vi "4Pi 4Pi Modes - Select Modes - BAK.vi"() -> ()   [LabVIEW 2016]
uses:
  4Pi 4Pi Modes - Controls/4Pi 4Pi Modes - Mirror Modes.ctl
  <vilib>/Utility/miscctls.llb/LVPointTypeDef.ctl
  Hardware Configuration/Hardware Configuration Controls/Standard Action.ctl
  4Pi 4Pi Modes - Controls/4Pi 4Pi Modes - Standard Action.ctl
  <userlib>/BMC/BMC.lvlib
panel:
  out "error out":errorcluster
  in  "Mirror Modes":T1
  in  "Flags":string
  in  "Change Modes":bool
  in  "Help":bool
  in  "Control mode":string(combo)="Single"
  in  "DM index":string(combo)="0"
  out "standard output":string
  out "standard error":string
  in  "Calling VI Ref":refnum<vi>
  in  "Exit":bool
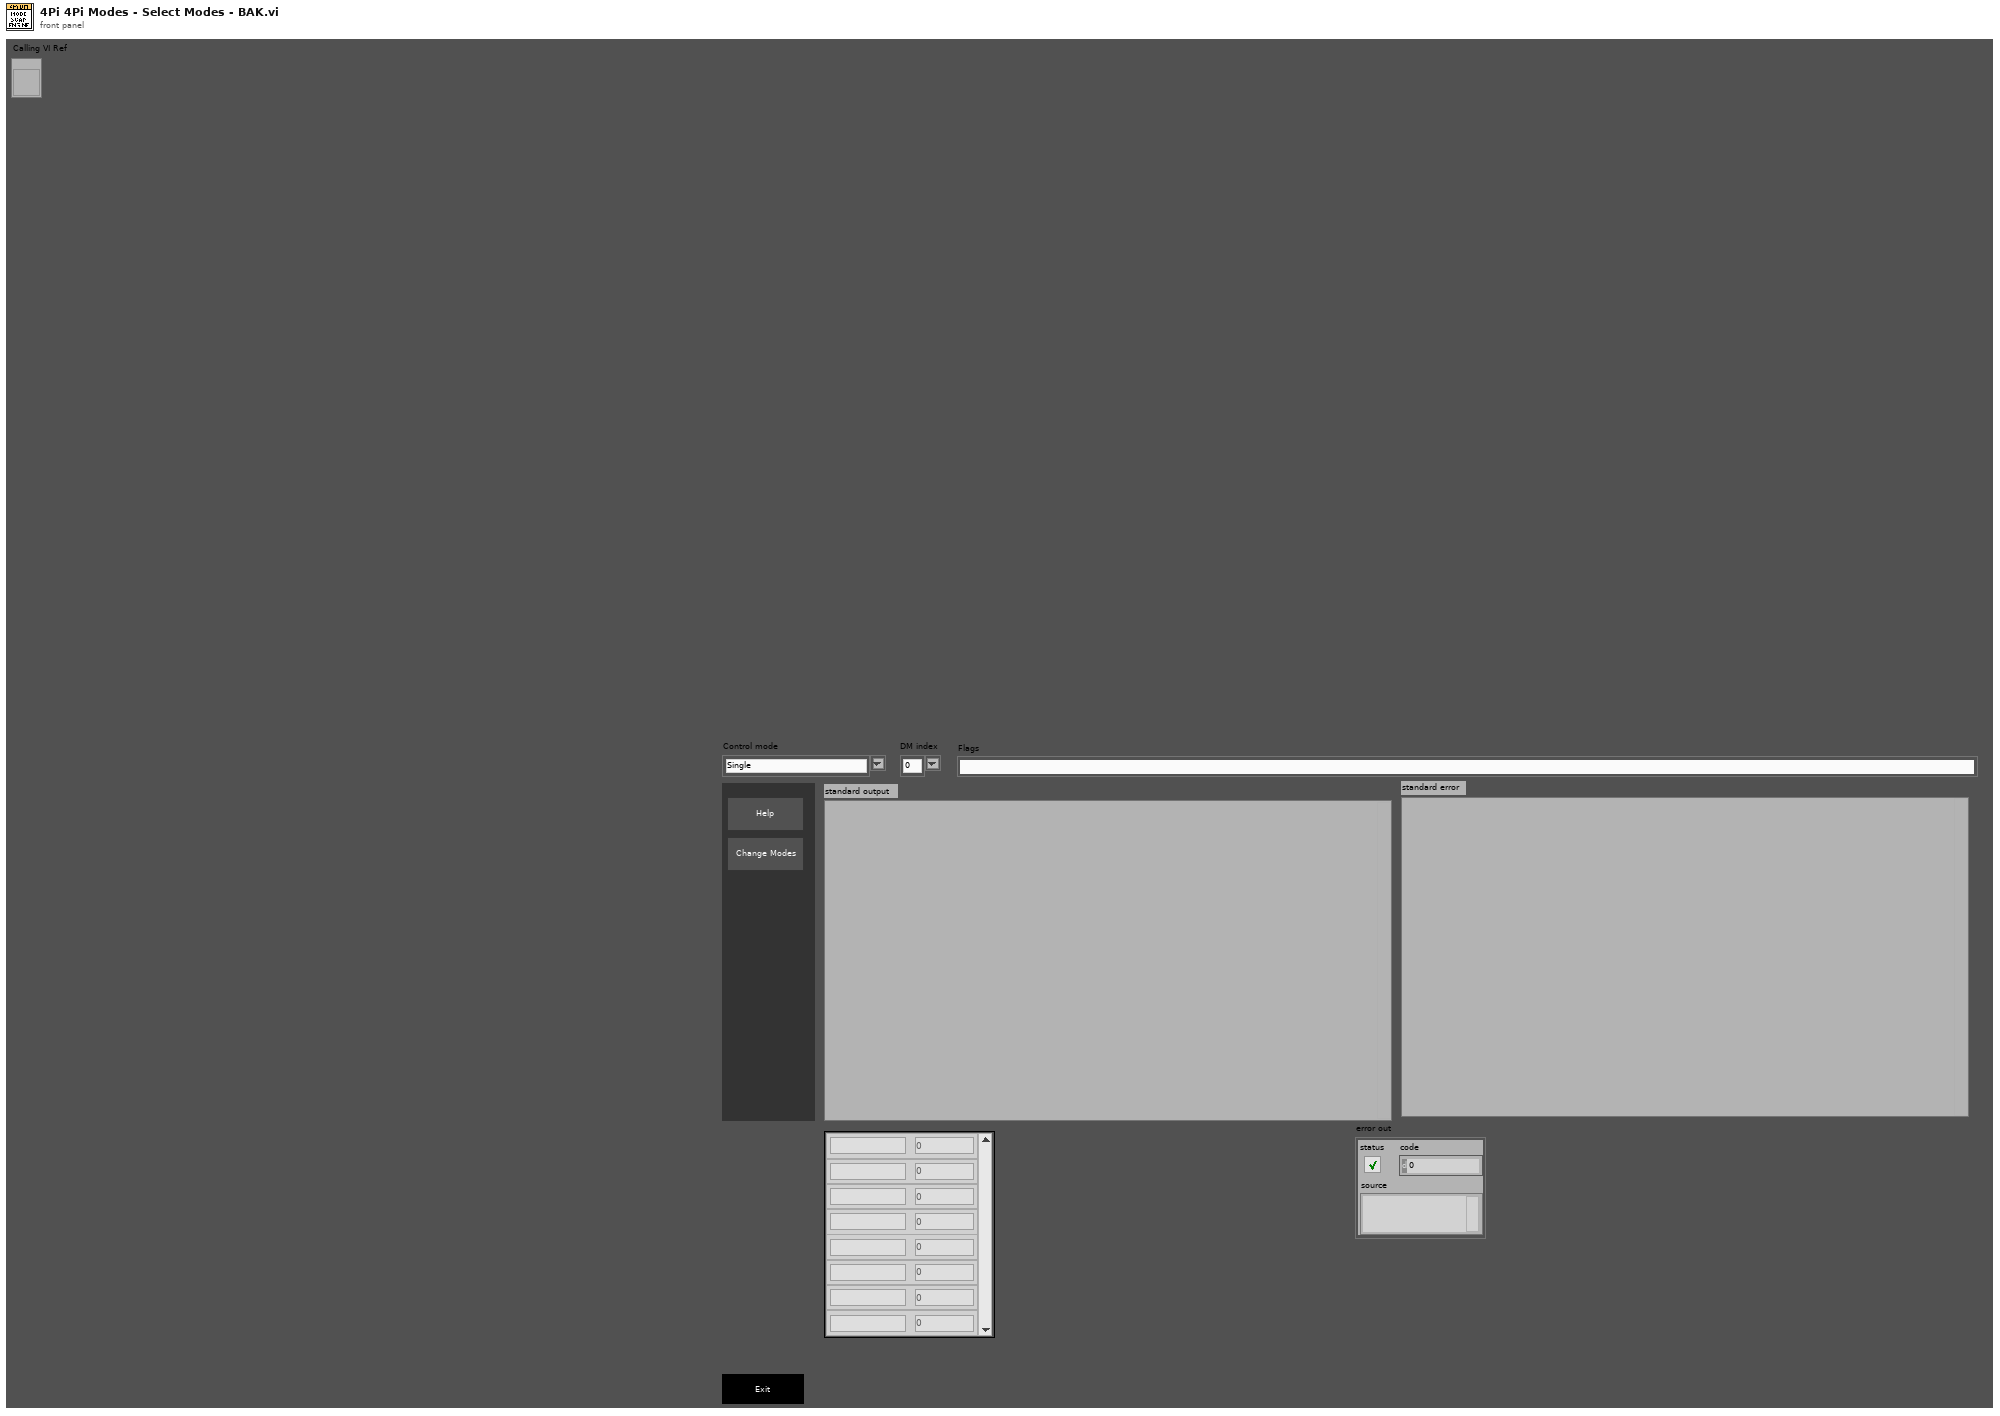
[diagram p1: front panel]
types:
  T1 = typedef "4Pi 4Pi Modes - Mirror Modes.ctl" = cluster{"Mode":string, "Amplitude":dbl}[]
  T2 = enum16{"Always On", "Always Off", "Off While Running"}
  T3 = typedef "LVPointTypeDef.ctl" = cluster{"Horizontal":i16, "Vertical":i16}
  T4 = typedef "LVRectTypeDef.ctl" = cluster{"Left":i16, "Top":i16, "Right":i16, "Bottom":i16}
  T5 = typedef "LVBoundsTypeDef.ctl" = cluster{"Width":u32, "Height":u32}
  T6 = typedef "Standard Action.ctl" = enum16{"Read", "Write"}
  T7 = typedef "4Pi 4Pi Modes - Standard Action.ctl" = enum16{"Read", "Write"}
  T8 = cluster{"type":i16, "ID":i16, "size":i32, "lutName":u64, "priv":u64}[]
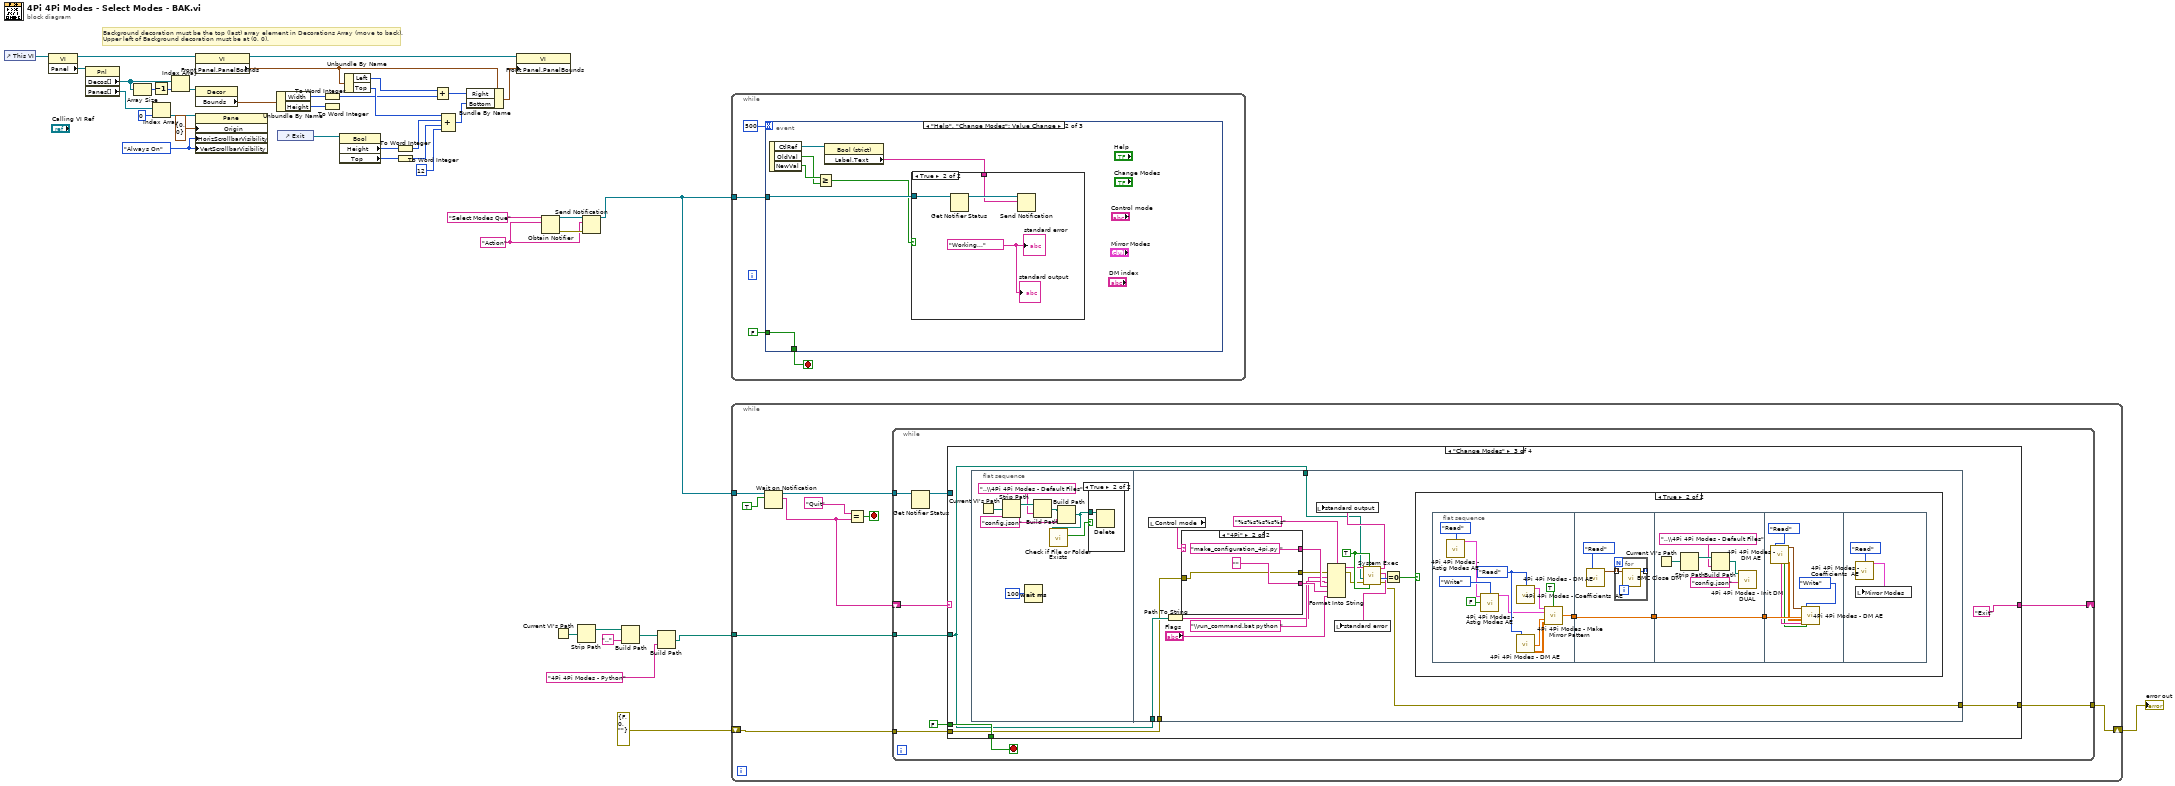
[diagram p0: block diagram]
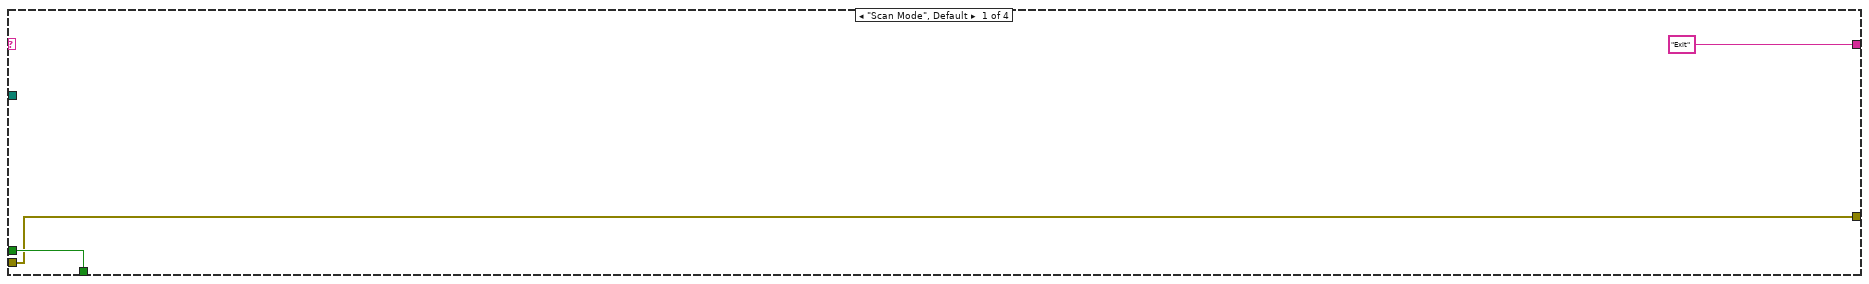
[diagram p2: hidden frame]
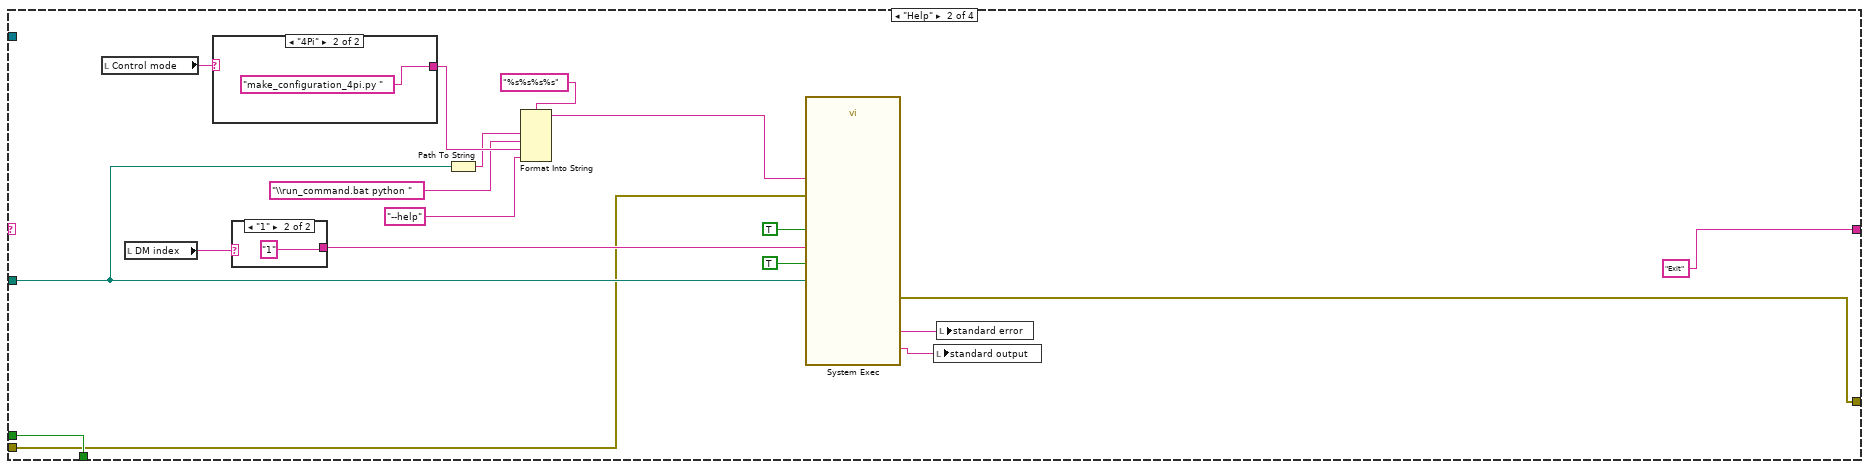
[diagram p3: hidden frame]
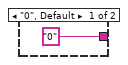
[diagram p4: hidden frame]
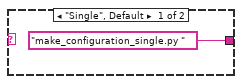
[diagram p5: hidden frame]
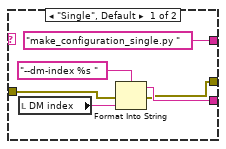
[diagram p8: hidden frame]
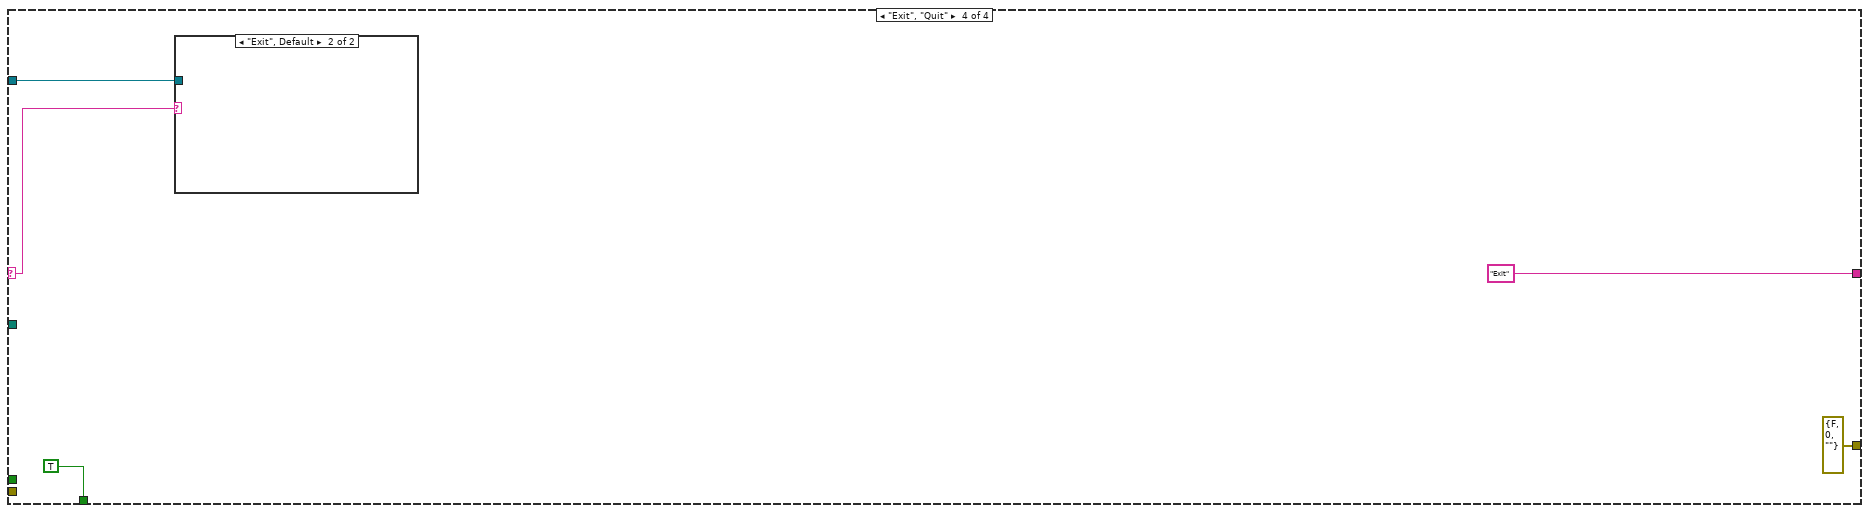
[diagram p9: hidden frame]
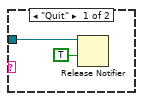
[diagram p10: hidden frame]
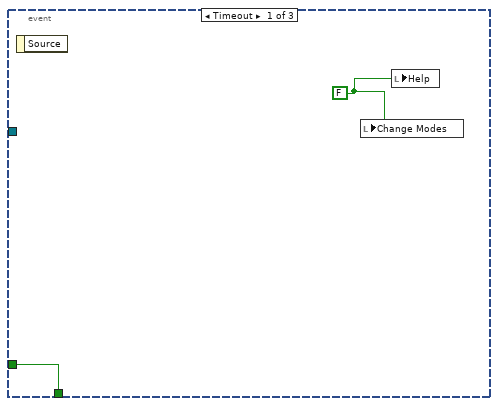
[diagram p11: hidden frame]
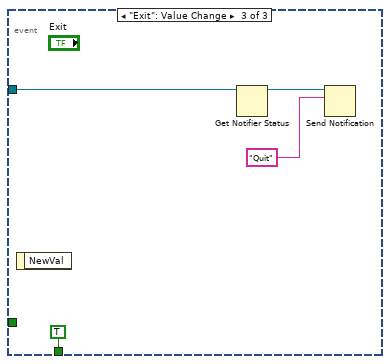
[diagram p13: hidden frame]
diagram:
  w9 = "Action" ("name (unnamed)")
  w25 = T2."Always On" ("Vertical Scrollbar Visibility")
  # "Background decoration must be the top (last) array element in Decorations Array (move to back).\nUpper left of Background decoration must be at (0, 0)."
  n1 = control-ref of="This VI"() -> (w17:refnum<vi>)
  n2 = property class="VI"(reference=w17) -> (reference out=w26:refnum<vi>, "Panel"=w18:refnum<vi>)  [unwired: 1 in, 1 out]
  n3 = property class="Pnl"(reference=w18) -> ("Decos[]"=w16:refnum<vi>[], "Panes[]"=w22:refnum<vi>[])  [unwired: 1 in, 2 out]
  n4 = Array Size(array=w16) -> (size(s)=w14:i32)
  n5 = Decrement(x=w14) -> (x-1=w15:i32)
  n6 = Index Array(array=w22, index=0) -> (element=w21:refnum<vi>)
  n7 = Index Array(array=w16, index=w15) -> (element=w24:refnum<vi>)
  n8 = property class="VI"(reference=w26) -> (reference out=w28:refnum<vi>, "Front Panel.PanelBounds"=w29:T4)  [unwired: 1 in, 1 out]
  n9 = property class="Decor"(reference=w24) -> ("Bounds"=w27:T5)  [unwired: 1 in, 2 out]
  n10 = property class="Pane"(reference=w21, "Origin"=T3 {"Horizontal"=0, "Vertical"=0}, "HorizScrollbarVisibility"=w25, "VertScrollbarVisibility"=w25) -> ()  [unwired: 1 in, 2 out]
  n11 = Unbundle By Name(w27) -> ("Width"=w32:u32, "Height"=w35:u32)
  n12 = control-ref of="Exit"() -> (w19:refnum<vi>)
  n13 = To Word Integer(number=w32) -> (16bit integer=w34:i16)
  n14 = To Word Integer(number=w35) -> ()  [unwired: 1 out]
  n15 = property class="Bool"(reference=w19) -> ("Height"=w37:u32, "Top"=w38:i32)  [unwired: 1 in, 2 out]
  n16 = Unbundle By Name(w29) -> ("Left"=w31:i16, "Top"=w42:i16)
  n17 = To Word Integer(number=w37) -> (16bit integer=w40:i16)
  n18 = To Word Integer(number=w38) -> (16bit integer=w41:i16)
  n19 = Add(x=w31, y=w34) -> (x+y=w33:i16)
  n20 = Compound Arithmetic op=ADD(w42, w40, w41, i16 12 ("y")) -> (w36:i16)
  n21 = Bundle By Name(cluster=w29, "Right"=w33, "Bottom"=w36) -> (w30:T4)
  n22 = property class="VI"(reference=w28, "Front Panel.PanelBounds"=w30) -> ()  [unwired: 1 in, 2 out]
  n23 = Obtain Notifier(name (unnamed)="Select Modes Que", notification data type=w9) -> (notifier out=w11:refnum<notifier>, error out=w12:errorcluster)  [unwired: 2 in, 1 out]
  n24 = Current VI's Path() -> (path=w7:path)
  n25 = Strip Path(path=w7) -> (stripped path=w6:path)  [unwired: 1 out]
  n26 = Send Notification(notification=w9, notifier=w11, error in (no error)=w12) -> (notifier out=w10:refnum<notifier>)  [unwired: 1 out]
  n27 = Build Path(base path=w6, name or relative path="..") -> (appended path=w4:path)
  n28 = Build Path(base path=w4, name or relative path="4Pi 4Pi Modes - Python") -> (appended path=w3:path)
  n29 = while {
    tunnel: w10 -> [w45]
    stop <- w43 stop-if-true
    n30 = event shown="[1] \"Help\", \"Change Modes\": Value Change" {
      selector: _ -> [_ _ _]
      dyn-events: _ -> [_ _ _]
      timeout: 500 -> [_ _ _]
      tunnel: w45 -> [_ w55 w62]
      tunnel: [w48 w54 TRUE] -> w43
      tunnel: FALSE -> [w48 w54 _]
      event Timeout {
        w47 = FALSE
        n31 = event-data() -> ()  [unwired: 1 in, 1 out]
        n32 = local write "Change Modes"(w47) -> ()
        n33 = local write "Help"(w47) -> ()
      }
      event "Help", "Change Modes": Value Change {
        n34 = event-data() -> ("CtlRef"=w53:refnum<vi>, "OldVal"=w50:bool, "NewVal"=w51:bool)  [unwired: 1 in]
        n35 = Greater Or Equal?(x=w51, y=w50) -> (x >= y?=w49:bool)
        n36 = property class="Bool (strict)"(reference=w53) -> ("Label.Text"=w52:string)  [unwired: 1 in, 2 out]
        n37 = case shown="True" w49 {
          tunnel: w55 -> [_ w58]
          tunnel: w52 -> [_ w56]
          frame False {
          }
          frame True {
            w57 = "Working..." ("standard error")
            n38 = Get Notifier Status(notifier=w58) -> (notifier out=w59:refnum<notifier>)  [unwired: 1 in, 4 out]
            n39 = Send Notification(notification=w56, notifier=w59) -> ()  [unwired: 1 in, 2 out]
            "standard error" <- w57
            "standard output" <- w57
          }
        }
      }
      event "Exit": Value Change {
        n40 = event-data() -> ()  [unwired: 1 in, 1 out]
        n41 = Get Notifier Status(notifier=w62) -> (notifier out=w63:refnum<notifier>)  [unwired: 1 in, 4 out]
        n42 = Send Notification(notification="Quit", notifier=w63) -> ()  [unwired: 1 in, 2 out]
      }
    }
  }
  n43 = while {
    tunnel: w10 -> [w72]
    tunnel: w3 -> [w66]
    shift-right: [w65] -> w1
    shift-left: errorcluster {"status"=FALSE, "code"=0, "source"=""} ("error in") -> [w64]
    stop <- w69 stop-if-true
    n44 = Wait on Notification(notifier=w72, ignore previous (F)=TRUE) -> (notifier out=w70:refnum<notifier>, notification=w67:string)  [unwired: 2 in, 2 out]
    n45 = Equal?(x="Quit" ("name (unnamed)"), y=w67) -> (x = y?=w69:bool)
    n46 = while {
      tunnel: w70 -> [w80]
      tunnel: w66 -> [w76]
      shift-right: [w75] -> _
      shift-left: w67 -> [w77]
      tunnel: [w74] -> w65
      tunnel: w64 -> [w73]
      stop <- w81 stop-if-true
      n47 = Get Notifier Status(notifier=w80) -> (notifier out=w79:refnum<notifier>)  [unwired: 1 in, 4 out]
      n48 = case shown="\"Change Modes\"" w77 {
        selector: w77 -> [_ _ _ w184]
        tunnel: [w84 w88 w111 TRUE] -> w81
        tunnel: w79 -> [_ _ _ w186]
        tunnel: FALSE -> [w84 w88 w111 _]
        tunnel: w76 -> [_ w89 w107 _]
        tunnel: ["Exit" ("name (unnamed)") "Exit" ("name (unnamed)") "Exit" ("name (unnamed)") "Exit" ("name (unnamed)")] -> w75
        tunnel: [w82 w85 w109 errorcluster {"status"=FALSE, "code"=0, "source"=""} ("error out")] -> w74
        tunnel: w73 -> [w82 w86 w108 _]
        frame "Scan Mode", Default {
        }
        frame "Help" {
          n49 = local read "Control mode"() -> (w94:string)
          n50 = local read "DM index"() -> (w101:string)
          n51 = case shown="\"4Pi\"" w94 {
            tunnel: ["make_configuration_single.py " "make_configuration_4pi.py "] -> w99
            frame "Single", Default {
            }
            frame "4Pi" {
            }
          }
          n52 = case shown="\"1\"" w101 {
            tunnel: ["0" ("name or relative path") "1" ("name or relative path")] -> w102
            frame "0", Default {
            }
            frame "1" {
            }
          }
          n53 = Path To String(path=w89) -> (string=w96:string)
          n54 = Format Into String(format string="%s%s%s%s", w96, "\\run_command.bat python " ("name or relative path"), w99, "--help" ("name or relative path")) -> (resulting string=w98:string)  [unwired: 2 in, 1 out]
          n55 = call <vilib>:"System Exec.vi"("run minimized? (F)"=TRUE, "wait until completion? (T)"=TRUE, "error in (no error)"=w86, "working directory"=w89, "standard input"=w102, "command line"=w98) -> ("error out"=w85:errorcluster, "standard error"=w92:string, "standard output"=w93:string)  [unwired: 2 in, 1 out]
          n56 = local write "standard output"(w93) -> ()
          n57 = local write "standard error"(w92) -> ()
        }
        frame "Change Modes" {
          n58 = flat-sequence {
            tunnel: w107 -> [w129]
            tunnel: [w123] -> w109
            tunnel: w108 -> [w122]
            tunnel: w107 -> [w121]
            frame #0 {
              n59 = Current VI's Path() -> (path=w118:path)
              n60 = Strip Path(path=w118) -> (stripped path=w119:path)  [unwired: 1 out]
              n61 = Wait (ms)(milliseconds to wait=u32 100) -> ()  [unwired: 1 out]
              n62 = Build Path(base path=w119, name or relative path="..\\4Pi 4Pi Modes - Default Files") -> (appended path=w116:path)
              n63 = Build Path(base path=w116, name or relative path="config.json") -> (appended path=w113:path)
              n64 = call <vilib>:"Check if File or Folder Exists.vi"("path"=w113) -> ("file or folder exists?"=w114:bool)  [unwired: 8 in, 2 out]
              n65 = case shown="True" w114 {
                tunnel: w113 -> [_ w120]
                frame False {
                }
                frame True {
                  n66 = Delete(path (use dialog)=w120) -> ()  [unwired: 4 in, 3 out]
                }
              }
            }
            frame #1 {
              w139 = TRUE ("run minimized? (F)")
              n67 = local read "Control mode"() -> (w130:string)
              n68 = Path To String(path=w129) -> (string=w132:string)
              n69 = case shown="\"4Pi\"" w130 {
                tunnel: ["make_configuration_single.py " "make_configuration_4pi.py "] -> w135
                tunnel: [w177 ""] -> w138
                tunnel: w122 -> [w175 w180]
                tunnel: [w174 w180] -> w125
                frame "Single", Default {
                  n70 = local read "DM index"() -> (w176:string)
                  n71 = Format Into String(format string="--dm-index %s ", error in=w175, w176) -> (resulting string=w177:string, error out=w174:errorcluster)  [unwired: 1 in]
                }
                frame "4Pi" {
                }
              }
              n72 = Format Into String(format string="%s%s%s%s%s", error in=w125, w132, "\\run_command.bat python " ("name or relative path"), w135, w138, "Flags") -> (resulting string=w134:string, error out=w124:errorcluster)  [unwired: 1 in]
              n73 = call <vilib>:"System Exec.vi"("run minimized? (F)"=w139, "wait until completion? (T)"=w139, "error in (no error)"=w124, "working directory"=w121, "command line"=w134) -> ("error out"=w123:errorcluster, "return code"=w136:i32, "standard error"=w127:string, "standard output"=w128:string)  [unwired: 3 in]
              n74 = local write "standard output"(w128) -> ()
              n75 = local write "standard error"(w127) -> ()
              n76 = Equal To 0?(x=w136) -> (x = 0?=w126:bool)
              n77 = case shown="True" w126 {
                frame False {
                }
                frame True {
                  n78 = flat-sequence {
                    tunnel: [w144] -> w142
                    tunnel: w142 -> [w156]
                    tunnel: [w156] -> w141
                    tunnel: w141 -> [w159]
                    tunnel: [w159] -> w140
                    tunnel: w140 -> [w168]
                    frame #0 {
                      w150 = 4Pi_4Pi_Modes_-_Standard_Action."Read" ("Action")
                      n79 = call "4Pi 4Pi Modes - Astig Modes AE.vi"("Action"=Standard_Action."Read") -> ("Coefficients Out"=w145:cluster{"Mode":string, "Amplitude":dbl}[])  [unwired: 13 in, 1 out]
                      n80 = call "4Pi 4Pi Modes - Astig Modes AE.vi"("Coefficients In"=w145, "Action"=Standard_Action."Write", "Enabled In"=FALSE) -> ("Coefficients Out"=w148:cluster{"Mode":string, "Amplitude":dbl}[])  [unwired: 11 in, 1 out]
                      n81 = call "4Pi 4Pi Modes - Coefficients  AE.vi"("Action"=w150) -> ("Coefficients Out"=w149:cluster{"Mode":string, "Amplitude":dbl}[])  [unwired: 14 in]
                      n82 = call "4Pi 4Pi Modes - DM AE.vi"("Action"=w150) -> ("Flats Out"=w147:dbl[], "Control Matrix Out"=w146:dbl[][])  [unwired: 14 in, 3 out]
                      n83 = call "4Pi 4Pi Modes - Make Mirror Pattern.vi"("Coefficients"=w149, "Flat On?"=TRUE, "Astig Coeffs"=w148, "Flats"=w147, "Control Matrix"=w146) -> ("Pixel Value U (-1 to 1)"=w144:dbl[])  [unwired: 9 in, 1 out]
                    }
                    frame #1 {
                      n84 = call "4Pi 4Pi Modes - DM AE.vi"("Action"=4Pi_4Pi_Modes_-_Standard_Action."Read") -> ("DM Handles Out"=w154:T8)  [unwired: 14 in, 4 out]
                      n85 = for {
                        tunnel: w154 -> [w158] mode=indexing
                        tunnel: [w157] -> _ mode=indexing
                        n86 = call <userlib>:"BMC Close DM.vi"("dmHandle"=w158) -> ("function return"=w157:i32)  [unwired: 9 in, 1 out]
                      }
                    }
                    frame #2 {
                      n87 = Current VI's Path() -> (path=w161:path)
                      n88 = Strip Path(path=w161) -> (stripped path=w162:path)  [unwired: 1 out]
                      n89 = Build Path(base path=w162, name or relative path="..\\4Pi 4Pi Modes - Default Files") -> (appended path=w164:path)
                      n90 = call "4Pi 4Pi Modes - Init DM DUAL.vi"("Config File"="config.json" ("name or relative path"), "Base File Path"=w164) -> ()  [unwired: 8 in, 2 out]
                    }
                    frame #3 {
                      n91 = call "4Pi 4Pi Modes - DM AE.vi"("Action"=4Pi_4Pi_Modes_-_Standard_Action."Read") -> ("Serials Out"=w166:string[], "No hardware Out"=w165:bool, "DM Handles Out"=w169:T8, "Control Matrix Out"=w167:dbl[][])  [unwired: 14 in, 1 out]
                      n92 = call "4Pi 4Pi Modes - DM AE.vi"("DM Handles"=w169, "Flats"=w168, "Control Matrix"=w167, "Serials"=w166, "Action"=4Pi_4Pi_Modes_-_Standard_Action."Write", "No hardware"=w165) -> ()  [unwired: 9 in, 5 out]
                    }
                    frame #4 {
                      n93 = call "4Pi 4Pi Modes - Coefficients  AE.vi"("Action"=4Pi_4Pi_Modes_-_Standard_Action."Read") -> ("Coefficients Out"=w172:cluster{"Mode":string, "Amplitude":dbl}[])  [unwired: 14 in]
                      n94 = local write "Mirror Modes"(w172) -> ()
                    }
                  }
                }
              }
            }
          }
        }
        frame "Exit", "Quit" {
          n95 = case shown="\"Exit\", Default" w184 {
            tunnel: w186 -> [w189 _]
            frame "Quit" {
              n96 = Release Notifier(notifier=w189, force destroy? (F)=TRUE) -> ()  [unwired: 1 in, 3 out]
            }
            frame "Exit", Default {
            }
          }
        }
      }
    }
  }
  "error out" <- w1
